vi "vms_acceptCommand_SetValue.vi"(8 "error in (no error)":errorcluster, 11 "command_SetValue_Ctl":T1) -> (0 "error out":errorcluster, 2 "function return":i32, 3 "command_SetValue_Ctl out":T1)   [LabVIEW 2016, in "SALLV_vms.lvlib"]
doc: "int vms_shm_acceptCommand_SetValueLV(vms_command_SetValueLV *command_SetValue_Ctl );"
uses:
  SALLV_vms.lvlib
  DataTypes/command_SetValue.ctl
  SALLV_vms.so
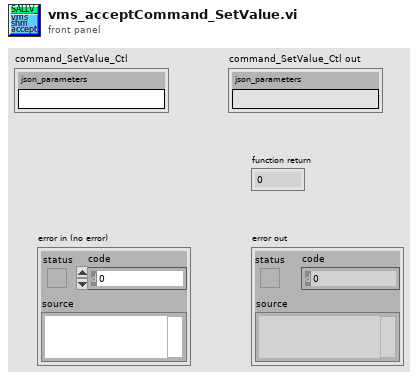
[diagram p1: front panel]
types:
  T1 = typedef "SALLV_vms.lvlib/command_SetValue.ctl" = cluster{"json_parameters":string}
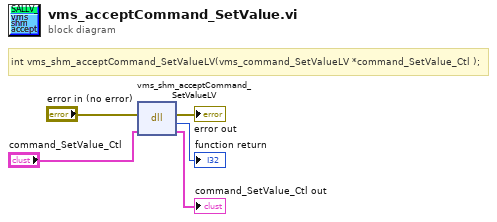
[diagram p0: block diagram]
diagram:
  # "int vms_shm_acceptCommand_SetValueLV(vms_command_SetValueLV *command_SetValue_Ctl );"
  n1 = dll-call lib="opt/CODE/SALLV_vms/SALLV_vms.*" fn="vms_shm_acceptCommand_SetValueLV"(error in="error in (no error)", "command_SetValue_Ctl"="command_SetValue_Ctl") -> (error out=→"error out":errorcluster, →"function return":i32, "command_SetValue_Ctl"=→"command_SetValue_Ctl out":T1)  [unwired: 2 in, 1 out]
